vi "Launch For G-CLI.vi"(8 "error in":errorcluster, 10 "Argument":string) -> (0 "error out":errorcluster)   [LabVIEW 2023, in "Adjust FP VIs.lvlib"]
uses:
  Adjust FP VIs.lvlib
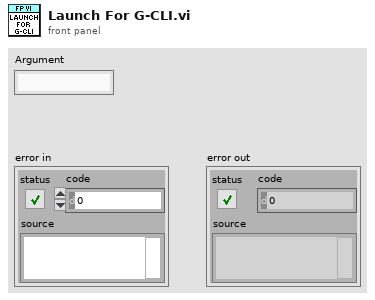
[diagram p1: front panel]
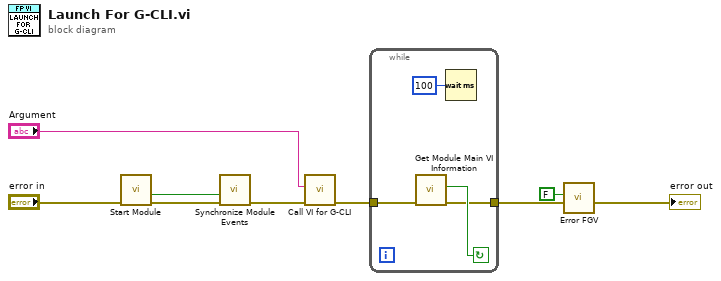
[diagram p0: block diagram]
diagram:
  n1 = call "Start Module.vi"("error in"="error in") -> ("error out"=w8:errorcluster, "Wait for Event Sync?"=w9:bool)  [unwired: 6 in, 3 out]
  n2 = call "Synchronize Module Events.vi"("error in"=w8, "Wait for Event Sync?"=w9) -> ("error out"=w7:errorcluster)  [unwired: 9 in]
  n3 = call "Call VI for G-CLI.vi"("error in"=w7, "Argument"="Argument") -> ("error out"=w4:errorcluster)  [unwired: 9 in]
  n4 = while {
    tunnel: w4 -> [w13]
    tunnel: [w10] -> w2
    stop <- w12 continue-if-true
    n5 = call "Get Module Main VI Information.vi"("error in"=w13) -> ("error out"=w10:errorcluster, "Is Module Running?"=w12:bool)  [unwired: 7 in, 2 out]
    n6 = Wait (ms)(milliseconds to wait=u32 100) -> ()  [unwired: 1 out]
  }
  n7 = call "Error FGV.vi"("error in"=w2, "Set?"=FALSE) -> ("error out"=→"error out":errorcluster)  [unwired: 9 in]
